vi "Check Linux Partition Size.vi"(8 "Error In":errorcluster, 10 "Warnings":T1[](array[typedef]), 11 "Install LV Data":T2={"SSH Session"=refnum, "Status Log"="", "Detailed Log"="", "Credentials"={"Hostname or IP"="192.168.7.2", "Username"="root", "Password"=""}, "Target Info"={"OS Version"="", "CPU"="", "Systemd Version"="", "Internet Access"=FALSE, "Device Type"="", "LV Installed Ver"="", "LV Available Ver"="", "LV Upgrade Available"=FALSE, "Hostname"="", "NIC Info"=[]}, "Reboot Required?"=FALSE}) -> (0 "Error Out":errorcluster, 2 "Warnings":T1[](array[typedef]), 3 "Install LV Data":T2={"SSH Session"=refnum, "Status Log"="", "Detailed Log"="", "Credentials"={"Hostname or IP"="192.168.7.2", "Username"="root", "Password"=""}, "Target Info"={"OS Version"="", "CPU"="", "Systemd Version"="", "Internet Access"=FALSE, "Device Type"="", "LV Installed Ver"="", "LV Available Ver"="", "LV Upgrade Available"=FALSE, "Hostname"="", "NIC Info"=[]}, "Reboot Required?"=FALSE})   [LabVIEW 2014, in "LMH-LINX.lvlib"]
uses:
  <vilib>/MakerHub/LINX/LMH-LINX.lvlib
  <vilib>/MakerHub/LINX/Private/Utilties/Target Management/Install LV Data.ctl
  C:/Program Files (x86)/National Instruments/LabVIEW 2014/vi.lib/MakerHub/LINX/Resources/Renci.SshNet.dll
  Resources/Renci.SshNet.dll
  <vilib>/MakerHub/LINX/Private/Utilties/Target Management/Target Info.ctl
  <vilib>/MakerHub/LINX/Private/Utilties/Target Management/NIC Info.ctl
  <vilib>/MakerHub/LINX/Private/Utilties/Target Management/NIC Mode.ctl
  <vilib>/MakerHub/LINX/Private/Utilties/Target Management/Target Compatibility Warnings.ctl
  <vilib>/regexp/Match Regular Expression.xnode
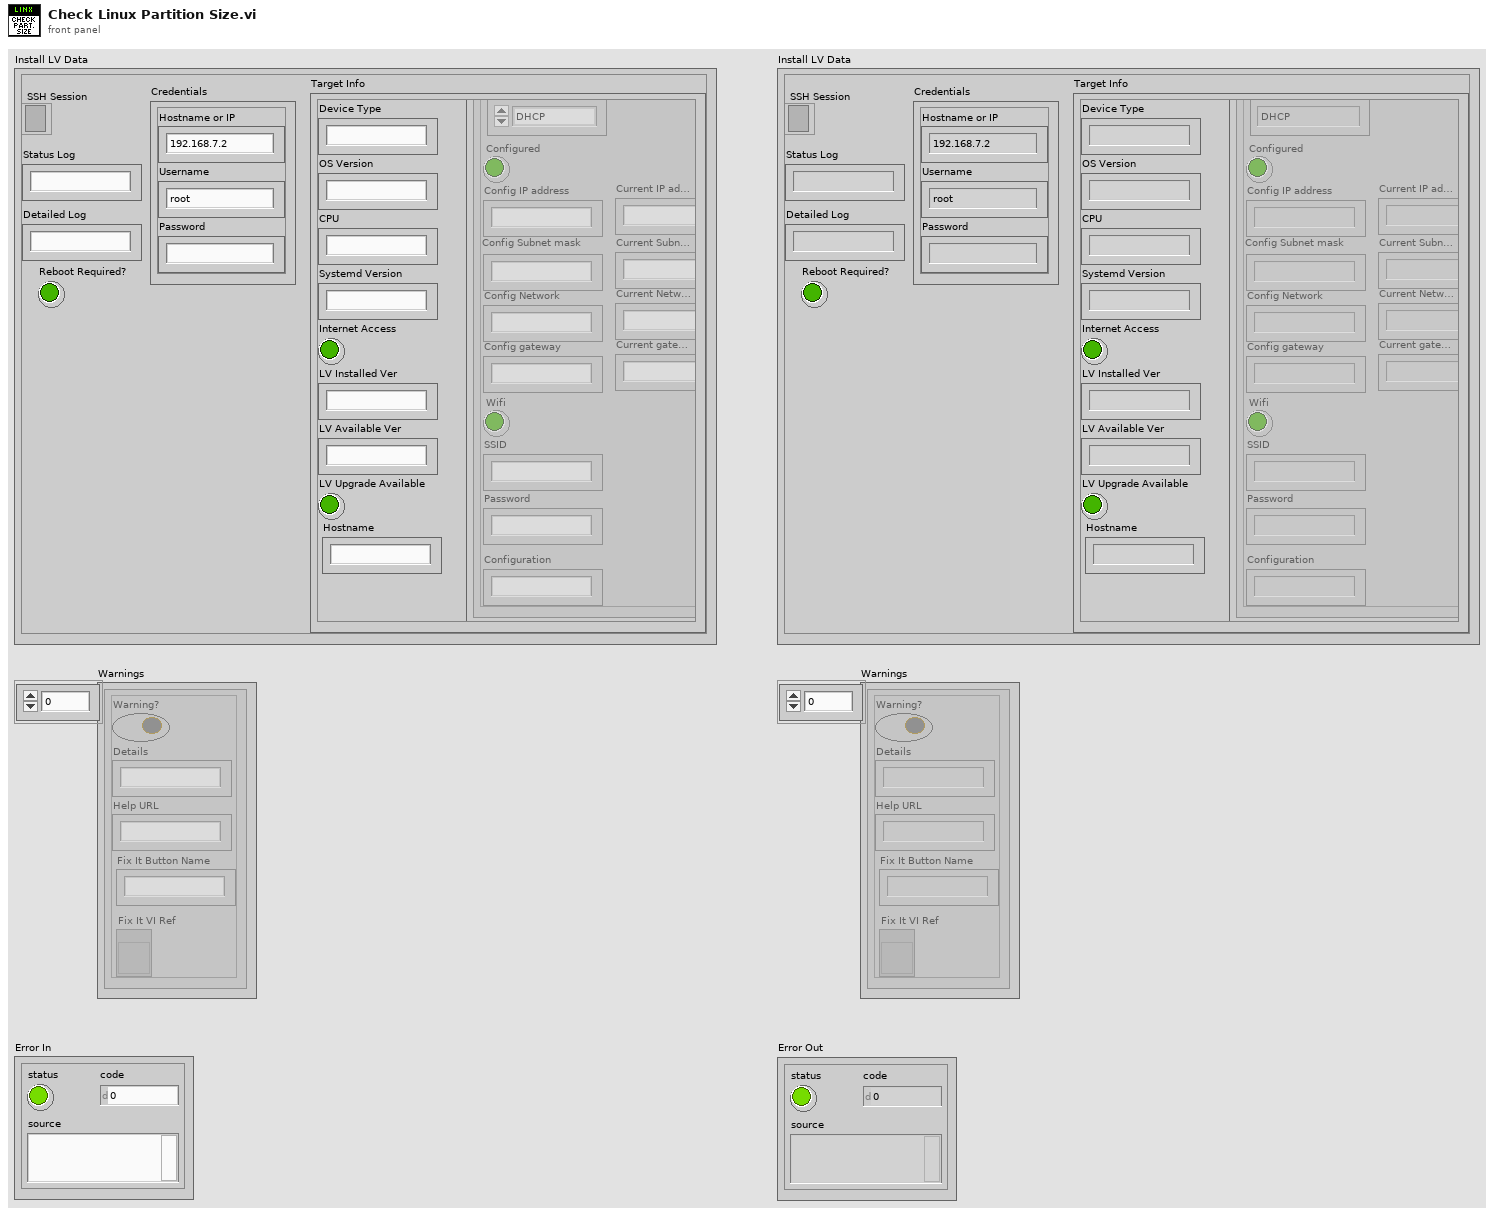
[diagram p1: front panel]
types:
  T1 = typedef "LMH-LINX.lvlib/Target Compatibility Warnings.ctl" = cluster{"Warning?":bool, "Details":string, "Help URL":string, "Fix It Button Name":string, "Fix It VI Ref":refnum<vi>}
  T2 = typedef "LMH-LINX.lvlib/Install LV Data.ctl" = cluster{"SSH Session":refnum<k24>, "Status Log":string, "Detailed Log":string, "Credentials":cluster{"Hostname or IP":string, "Username":string, "Password":string}, "Target Info":T3, "Reboot Required?":bool}
  T3 = typedef "LMH-LINX.lvlib/Target Info.ctl" = cluster{"OS Version":string, "CPU":string, "Systemd Version":string, "Internet Access":bool, "Device Type":string, "LV Installed Ver":string, "LV Available Ver":string, "LV Upgrade Available":bool, "Hostname":string, "NIC Info":T4[]}
  T4 = typedef "LMH-LINX.lvlib/NIC Info.ctl" = cluster{"Name":string, "NIC Mode":T5, "Configured":bool, "Config IP address":string, "Config Subnet mask":string, "Config Network":string, "Config gateway":string, "Wifi":bool, "SSID":string, "Password":string, "Configuration":string, "Current IP address":string, "Current Subnet mask":string, "Current gateway":string, "Current Network":string}
  T5 = typedef "LMH-LINX.lvlib/NIC Mode.ctl" = enum16{"DHCP", "Static", "Loopback"}
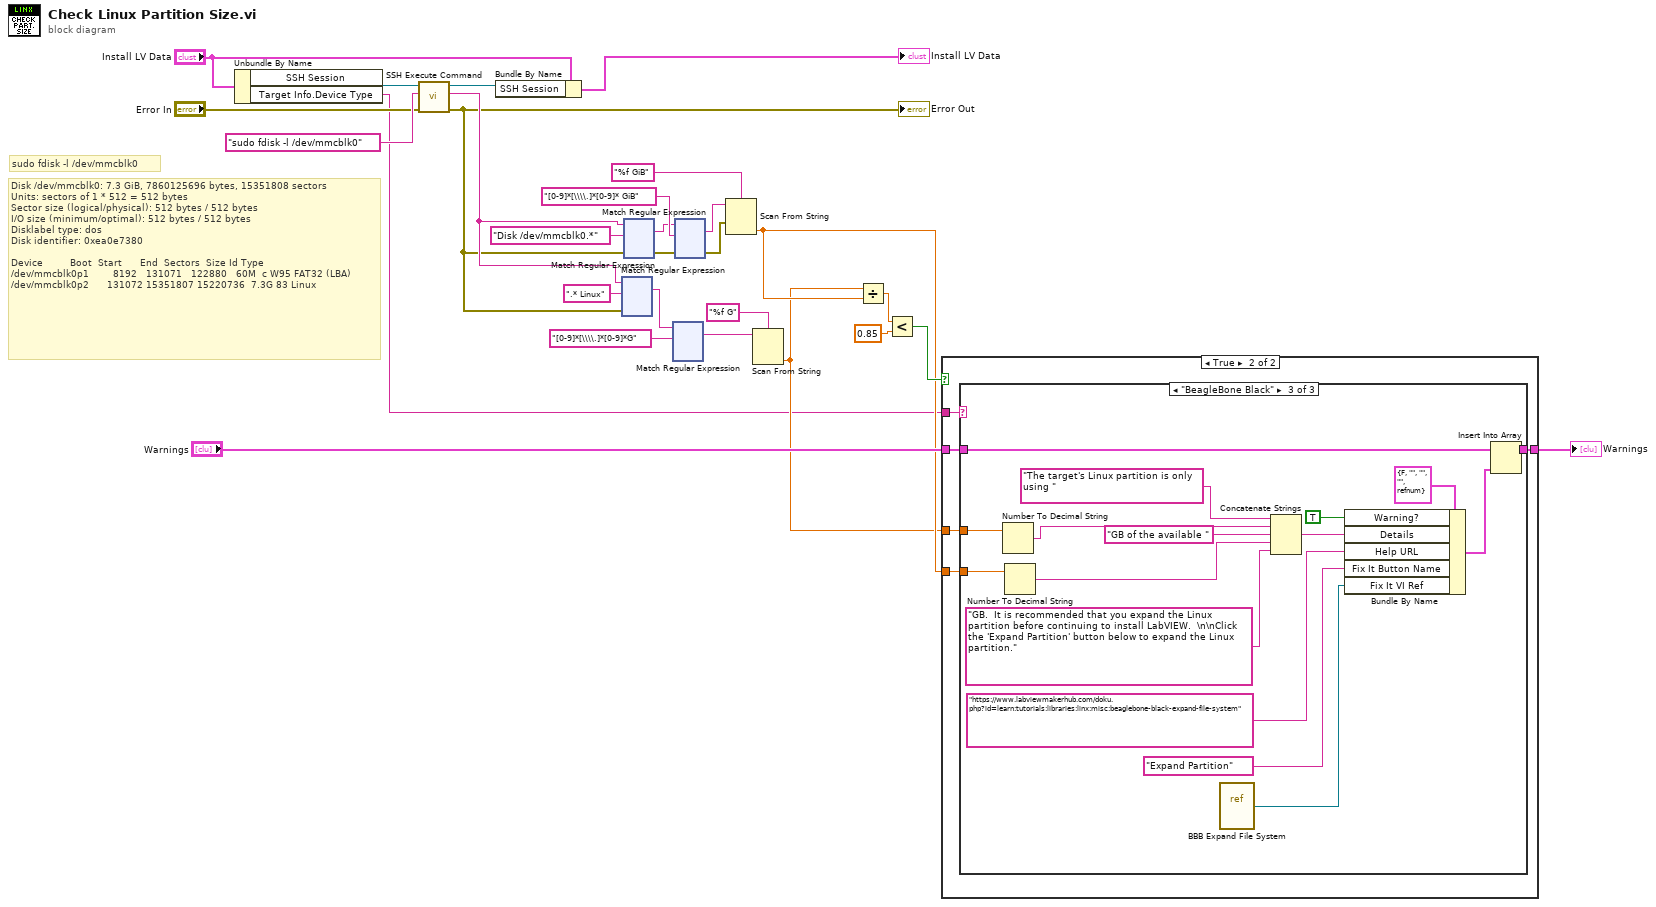
[diagram p0: block diagram]
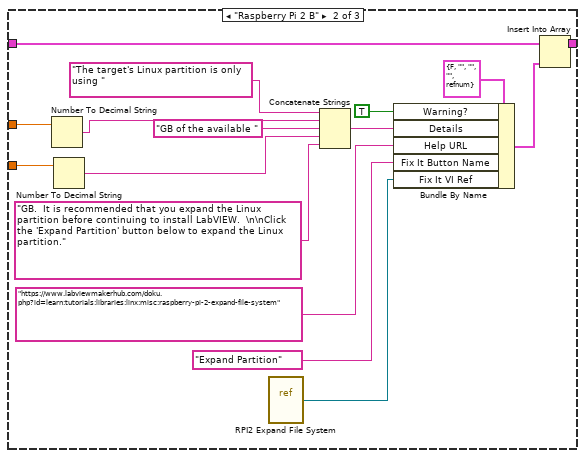
[diagram p4: hidden frame]
diagram:
  # "sudo fdisk -l /dev/mmcblk0"
  # "Disk /dev/mmcblk0: 7.3 GiB, 7860125696 bytes, 15351808 sectors\nUnits: sectors of 1 * 512 = 512 bytes\nSector size (logical/physical): 512 bytes / 512 bytes\nI/O size (minimum/optimal): 512 bytes / 512 bytes\nDisklabel type: dos\nDisk identifier: 0xea0e7380\n\nDevice         Boot  Start      End  Sectors  Size Id Type\n/dev/mmcblk0p1        8192   131071   122880   60M  c W95 FAT32 (LBA)\n/dev/mmcblk0p2      131072 15351807 15220736  7.3G 83 Linux"
  n1 = Unbundle By Name("Install LV Data") -> ("SSH Session"=w28:refnum<k24>, "Target Info.Device Type"=w2:string)
  n2 = call <vilib>:"SSH Execute Command.vi"("Error In"="Error In", "Command"="sudo fdisk -l /dev/mmcblk0", "SSH Session"=w28) -> ("Error Out"=w1:errorcluster, "Std Out"=w12:string, "SSH Session"=w25:refnum<k24>)  [unwired: 6 in]
  "Error Out" <- w1
  n3 = Bundle By Name(cluster="Install LV Data", "SSH Session"=w25) -> (→"Install LV Data":T2)
  n4 = xnode "Match Regular Expression"("input string"=w12, "regular expression"=".* Linux" ("String"), "error in"=w1) -> ("whole match"=w16:string)  [unwired: 3 in, 4 out]
  n5 = xnode "Match Regular Expression"("input string"=w12, "regular expression"="Disk /dev/mmcblk0.*" ("String"), "error in"=w1) -> ("whole match"=w18:string, "error out"=w22:errorcluster)  [unwired: 3 in, 3 out]
  n6 = xnode "Match Regular Expression"("input string"=w16, "regular expression"="[0-9]*[\\\\.]*[0-9]*G" ("String")) -> ("whole match"=w14:string)  [unwired: 4 in, 4 out]
  n7 = xnode "Match Regular Expression"("input string"=w18, "regular expression"="[0-9]*[\\\\.]*[0-9]* GiB" ("String"), "error in"=w22) -> ("whole match"=w19:string, "error out"=w9:errorcluster)  [unwired: 3 in, 3 out]
  n8 = Scan From String(format string="%f GiB", input string=w19, error in=w9) -> (output 1=w5:dbl)  [unwired: 2 in, 3 out]
  n9 = Scan From String(format string="%f G", input string=w14) -> (output 1=w4:dbl)  [unwired: 3 in, 3 out]
  n10 = Divide(x=w4, y=w5) -> (x/y=w11:dbl)
  n11 = Less?(x=w11, y=0.85) -> (x < y?=w6:bool)
  n12 = case shown="True" w6 {
    tunnel: "Warnings" -> [w29 w34]
    tunnel: [w29 w33] -> w7
    tunnel: w4 -> [_ w32]
    tunnel: w5 -> [_ w31]
    tunnel: w2 -> [_ w30]
    frame False {
    }
    frame True {
      n13 = case shown="\"BeagleBone Black\"" w30 {
        tunnel: w34 -> [w35 w46 w62]
        tunnel: [w35 w45 w61] -> w33
        tunnel: w32 -> [_ w44 w60]
        tunnel: w31 -> [_ w38 w54]
        frame "False", Default {
        }
        frame "Raspberry Pi 2 B" {
          n14 = Number To Decimal String(number=w44) -> (decimal integer string=w43:string)  [unwired: 1 in]
          n15 = Number To Decimal String(number=w38) -> (decimal integer string=w41:string)  [unwired: 1 in]
          n16 = vi-ref <vilib>:"RPI2 Expand File System.vi"() -> (w36:refnum<vi>)
          n17 = Concatenate Strings("The target's Linux partition is only using ", w43, "GB of the available " ("string"), w41, "GB.  It is recommended that you expand the Linux partition before continuing to install LabVIEW.  \n\nClick the 'Expand Partition' button below to expand the Linux partition." ("string")) -> (w47:string)
          n18 = Bundle By Name(cluster=T1 {"Warning?"=FALSE, "Details"="", "Help URL"="", "Fix It Button Name"="", "Fix It VI Ref"=refnum} ("Target Compatibility Warnings"), "Warning?"=TRUE ("Can Continue?"), "Details"=w47, "Help URL"="https://www.labviewmakerhub.com/doku.php?id=learn:tutorials:libraries:linx:misc:raspberry-pi-2-expand-file-system" ("string"), "Fix It Button Name"="Expand Partition" ("string"), "Fix It VI Ref"=w36) -> (w48:T1)
          n19 = Insert Into Array(array=w46, new element=w48) -> (w45:T1[])  [unwired: 1 in]
        }
        frame "BeagleBone Black" {
          n20 = Number To Decimal String(number=w60) -> (decimal integer string=w59:string)  [unwired: 1 in]
          n21 = Number To Decimal String(number=w54) -> (decimal integer string=w57:string)  [unwired: 1 in]
          n22 = vi-ref <vilib>:"BBB Expand File System.vi"() -> (w52:refnum<vi>)
          n23 = Concatenate Strings("The target's Linux partition is only using ", w59, "GB of the available " ("string"), w57, "GB.  It is recommended that you expand the Linux partition before continuing to install LabVIEW.  \n\nClick the 'Expand Partition' button below to expand the Linux partition." ("string")) -> (w63:string)
          n24 = Bundle By Name(cluster=T1 {"Warning?"=FALSE, "Details"="", "Help URL"="", "Fix It Button Name"="", "Fix It VI Ref"=refnum} ("Target Compatibility Warnings"), "Warning?"=TRUE ("Can Continue?"), "Details"=w63, "Help URL"="https://www.labviewmakerhub.com/doku.php?id=learn:tutorials:libraries:linx:misc:beaglebone-black-expand-file-system" ("string"), "Fix It Button Name"="Expand Partition" ("string"), "Fix It VI Ref"=w52) -> (w64:T1)
          n25 = Insert Into Array(array=w62, new element=w64) -> (w61:T1[])  [unwired: 1 in]
        }
      }
    }
  }
  "Warnings" <- w7
